vi "Configure Laser Power.vi"(7 "Ignore Errors":bool, 8 "error in (no error)":errorcluster, 10 "Laser Power":bool, 11 "VISA resource name":refnum<visa-resource-name>) -> (0 "error out":errorcluster, 3 "VISA resource name out":refnum<visa-resource-name>)   [LabVIEW 2011, in "Hokuyo URG Series.lvlib"]
doc: "This VI turns the laser on and off. By default the laser is turned on when the VISA session is opened in Initialize.vi and turned off when the VISA session is closed in Close.vi."
uses:
  Hokuyo URG Series.lvlib
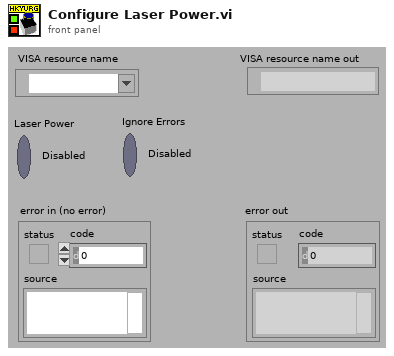
[diagram p1: front panel]
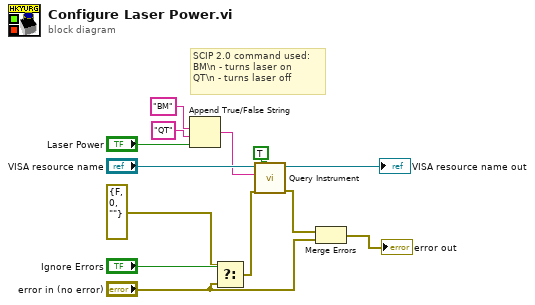
[diagram p0: block diagram]
diagram:
  # "SCIP 2.0 command used:\nBM\\n - turns laser on\nQT\\n - turns laser off"
  n1 = Append True/False String(1:"Laser Power", 2:"QT" ("false string"), 3:"BM" ("true string")) -> (0:w9:string)  [unwired: 1 out]
  n2 = Select(t=errorcluster {"status"=FALSE, "code"=0, "source"=""} ("error in (no error) 2"), s="Ignore Errors", f="error in (no error)") -> (s? t:f=w4:errorcluster)
  n3 = call "Query Instrument.vi"("Error Query (Enabled)"=TRUE, "error in"=w4, "Command"=w9, "VISA Resource Name"="VISA resource name") -> ("error out"=w3:errorcluster, "VISA Resource Name Out"=→"VISA resource name out":refnum<visa-resource-name>)  [unwired: 5 in, 1 out]
  n4 = Merge Errors(w3, "error in (no error)") -> (→"error out":errorcluster)
